vi "poly_control_signalling_write_multi_1.vi"(6 "mode (Sgnl)":T1(ring)=enum."Val(Sgnl)", 8 "error in (no error)":errorcluster, 9 "values":variant[](array[variant]), 10 "control names":string[](array[string]), 11 "vi reference":refnum<vi>) -> (0 "error out":errorcluster, 2 "control refs":refnum<vi>[](array[refnum]), 3 "vi reference out":refnum<vi>, 4 "found?":bool[](array[boolean]))   [LabVIEW 2015]
uses:
  poly_control_ref_from_name_multi.vi
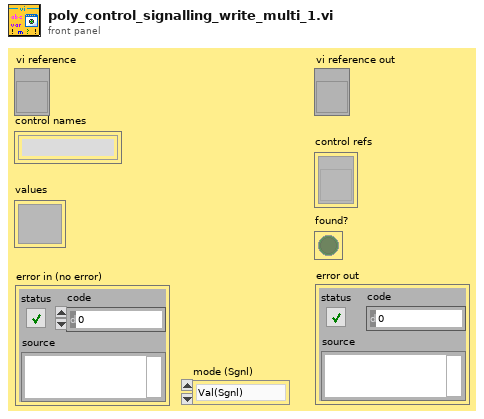
[diagram p1: front panel]
types:
  T1 = enum16{"Val", "Val(Sgnl)", "Val(Undo)", "Method"}
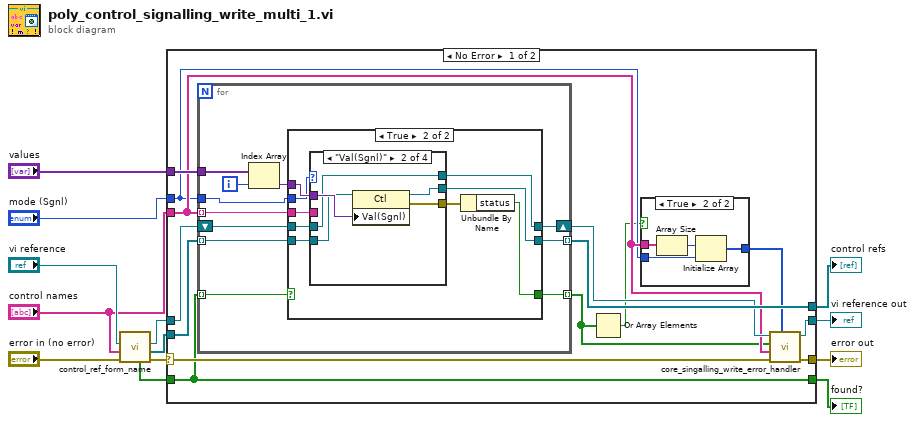
[diagram p0: block diagram]
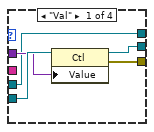
[diagram p4: hidden frame]
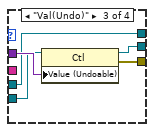
[diagram p5: hidden frame]
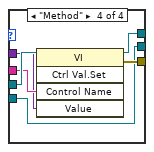
[diagram p6: hidden frame]
diagram:
  n1 = call-poly "control_ref_form_name.vi"("error in (no error)"="error in (no error)", "control names"="control names", "vi ref"="vi reference") -> ("error out"=w3:errorcluster, "ctrl refs"=w9:refnum<vi>[], "vi ref dup"=w8:refnum<vi>, "found?"=w4:bool[])  [unwired: 5 in]
  n2 = case shown="No Error" w3 {
    selector: w3 -> [w23 w79]
    tunnel: "mode (Sgnl)" -> [w17 _]
    tunnel: [w20 w78] -> w12
    tunnel: w9 -> [w27 w77]
    tunnel: w8 -> [w26 w78]
    tunnel: "control names" -> [w18 _]
    tunnel: "values" -> [w25 _]
    tunnel: [w24 w77] -> w5
    tunnel: w4 -> [w19 w76]
    tunnel: [w22 w79] -> w2
    tunnel: [w19 w76] -> w1
    frame No Error {
      n3 = for {
        tunnel: w17 -> [w42]
        tunnel: [w41] -> w24 mode=indexing
        tunnel: w27 -> [w34] mode=indexing
        tunnel: w18 -> [w37] mode=indexing
        shift-right: [w40] -> w21
        shift-left: w26 -> [w39]
        tunnel: w25 -> [w36]
        tunnel: w19 -> [w33] mode=indexing
        tunnel: [w32] -> w16 mode=indexing
        i -> [w38]
        n4 = Index Array(array=w36, index=w38) -> (element=w35:variant)
        n5 = case shown="True" w33 {
          selector: w33 -> [w43 _]
          tunnel: w35 -> [_ w54]
          tunnel: w42 -> [_ w53]
          tunnel: [w44 w52] -> w41
          tunnel: [w45 w51] -> w40
          tunnel: w37 -> [_ w50]
          tunnel: w39 -> [w45 w49]
          tunnel: w34 -> [w44 w48]
          tunnel: [w43 w46] -> w32
          frame False {
          }
          frame True {
            n6 = case shown="\"Val(Sgnl)\"" w53 {
              tunnel: w48 -> [w59 w61 w65 w73]
              tunnel: w54 -> [w58 w64 w69 w70]
              tunnel: [w57 w63 w66 w74] -> w47
              tunnel: [w56 w62 w68 w73] -> w52
              tunnel: w49 -> [w55 w60 w67 w75]
              tunnel: [w55 w60 w67 w72] -> w51
              tunnel: w50 -> [_ _ _ w71]
              frame "Val" {
                n7 = property class="Ctl"(reference=w59, "Value"=w58) -> (reference out=w56:refnum<vi>, error out=w57:errorcluster)  [unwired: 1 in]
              }
              frame "Val(Sgnl)" {
                n8 = property class="Ctl"(reference=w61, "Val(Sgnl)"=w64) -> (reference out=w62:refnum<vi>, error out=w63:errorcluster)  [unwired: 1 in]
              }
              frame "Val(Undo)" {
                n9 = property class="Ctl"(reference=w65, "Value (Undoable)"=w69) -> (reference out=w68:refnum<vi>, error out=w66:errorcluster)  [unwired: 1 in]
              }
              frame "Method" {
                n10 = invoke class="VI" method="Ctrl Val.Set"(reference=w75, "Control Name"=w71, "Value"=w70) -> (reference out=w72:refnum<vi>, error out=w74:errorcluster)  [unwired: 2 in, 3 out]
              }
            }
            n11 = Unbundle By Name(w47) -> ("status"=w46:bool)
          }
        }
      }
      n12 = Or Array Elements(Boolean array=w16) -> (logical OR=w15:bool)
      n13 = case shown="True" w15 {
        tunnel: w18 -> [_ w30]
        tunnel: w17 -> [_ w29]
        tunnel: [_ w28] -> w14
        frame False {
        }
        frame True {
          n14 = Array Size(array=w30) -> (size(s)=w31:i32)
          n15 = Initialize Array(w31, w29) -> (w28:i32[])
        }
      }
      n16 = call "core_singalling_write_error_handler.vi"("modes (Sgnl)"=w14, "error in"=w23, "control names"=w18, "error?"=w16, "vi ref"=w21) -> ("error out"=w22:errorcluster, "vi ref dup"=w20:refnum<vi>)  [unwired: 5 in]
    }
    frame Error {
    }
  }
  "error out" <- w2
  "vi reference out" <- w12
  "found?" <- w1
  "control refs" <- w5
